vi "Set Channel Function Coefficient.vi"(6 "Coefficient value":dbl, 8 "error in (no error)":errorcluster, 9 "Coefficient":u16(ring) items=["A", "B", "C", "D", "X1", "X2", "Y1", "Y2"], 10 "Channel":u16(ring) items=["A1"=0, "A2"=1, "A3"=2, "A4"=3, "A5"=4, "A6"=5, "A7"=6, "A8"=7, "A9"=8, "A10"=9, "K1"=200, "K2"=201, "K3"=202, "K4"=203, "FA1"=204, "FA2"=205, "FA3"=206, "FA4"=207], 11 "VISA resource name":refnum<visa-resource-name>) -> (0 "error out":errorcluster, 3 "VISA resource name out":refnum<visa-resource-name>)   [LabVIEW 2017, in "Sefram DAS220.lvlib"]
doc: "Setup coefficient for a channel function."
uses:
  <instrlib>/Sefram DAS220/Sefram DAS220.lvlib
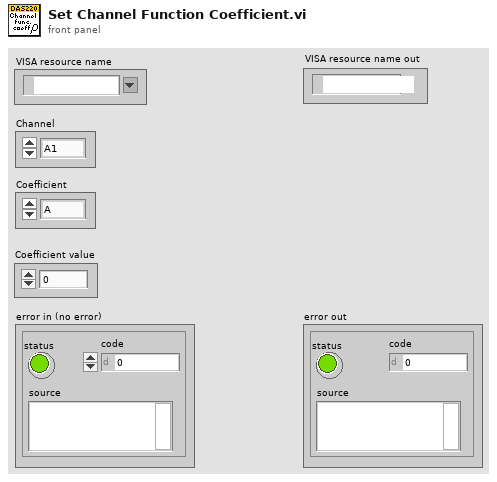
[diagram p1: front panel]
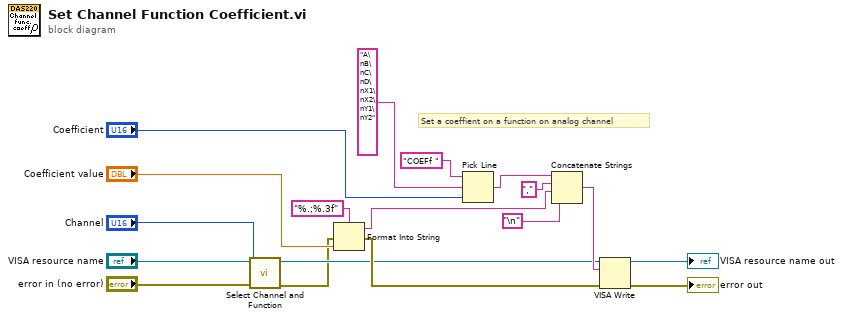
[diagram p0: block diagram]
diagram:
  # "Set a coeffient on a function on analog channel"
  n1 = call <instrlib>:"Select Channel and Function.vi"("error in (no error)"="error in (no error)", "Channel"="Channel", "VISA resource name"="VISA resource name") -> ("error out"=w3:errorcluster, "VISA resource name out"=w5:refnum<visa-resource-name>)  [unwired: 7 in]
  n2 = Format Into String(format string="%.;%.3f", error in=w3, "Coefficient value") -> (resulting string=w9:string, error out=w11:errorcluster)  [unwired: 1 in]
  n3 = Pick Line(string ("")="COEFf " ("string"), multi-line string="A\nB\nC\nD\nX1\nX2\nY1\nY2", line index="Coefficient") -> (output string=w14:string)
  n4 = Concatenate Strings(w14, "," ("string"), w9, "\n") -> (w18:string)
  n5 = VISA Write(VISA resource name=w5, write buffer=w18, error in (no error)=w11) -> (VISA resource name out=→"VISA resource name out":refnum<visa-resource-name>, error out=→"error out":errorcluster)  [unwired: 1 out]
